vi "Calc - P1P2.vi"(10 "P1":dbl, 11 "P2":dbl) -> (2 "RP1P2":dbl, 3 "P1P2":dbl)   [LabVIEW 2018, in "Controller (Host).lvlib"]
uses:
  Controller (Host).lvlib
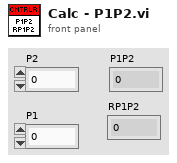
[diagram p1: front panel]
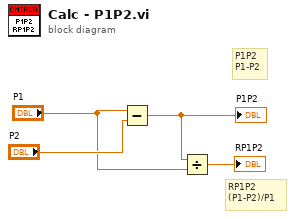
[diagram p0: block diagram]
diagram:
  # "RP1P2\n(P1-P2)/P1"
  # "P1P2\nP1-P2"
  n1 = Subtract(x="P1", y="P2") -> (x-y=w3:dbl)
  "P1P2" <- w3
  n2 = Divide(x=w3, y="P1") -> (x/y=→"RP1P2":dbl)
